vi "XML - Get relative RT Driver VI path.vi"(7 "Target Type (Windows)":T1, 10 "CD Template":refnum<class "NIVS_CD Template.lvclass">, 11 "Project Name":string) -> (3 "Relative RT Driver VI path":path)   [LabVIEW 2020, in "NIVS_Consolidated_CDW_MetaDataObj.lvclass"]
doc: "Create the relative path for the RT Driver VI inside the Configuration LLB based on the name and execution mode of the new custom device."
uses:
  NIVS_Consolidated_CDW_MetaDataObj.lvclass
  Build Spec Engine.ctl
  CD Engine lvlib.ctl
  Template Classes/NIVS_PPLCD Template/NIVS_PPLCD Template.lvclass
  Template Classes/NIVS_CD Template/NIVS_CD Template.lvclass
  Build Spec Engine.vi
  CD Engine lvlib.vi
  Target Type.ctl
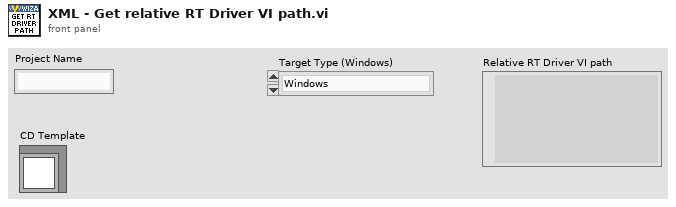
[diagram p1: front panel]
types:
  T1 = typedef "NIVS_Consolidated_CDW_MetaDataObj.lvclass/Target Type.ctl" = enum16{"Windows", "Linux x64"}
  T2 = typedef "NIVS_Consolidated_CDW_MetaDataObj.lvclass/CD Engine lvlib.ctl" = enum16{"LibraryFileName", "LibraryFolderName", "Engine.FolderName", "Engine.Init.FolderName", "Engine.Run.FolderName", "Engine.Shutdown.FolderName", "Types.FolderName", "Engine.RT Driver VI.TemplatePath", "Engine.RT Driver VI.FileName", "Engine.PPL.RT Driver VI_InlineAsync.FileName", "Engine.RTStateVariables.Name", "Engine.PPL.RTStateVariables.Name", "Engine.RTStateVariables.Name.NoExtension", "Engine.Async.NameExtension", "Engine.Async.TemplateName", "Engine.PPL.Async.TemplateName", "Engine.PPL.Async.InitVSGlobals.Name", "Engine.PPL.RT Driver VI_Inline.FileName"}
  T3 = typedef "NIVS_Consolidated_CDW_MetaDataObj.lvclass/Build Spec Engine.ctl" = enum16{"Destinations.LLBWindowsFileName", "Destinations.LLBLinux64FileName", "Destinations.PPLWindowsFileName", "Destinations.PPLLinux64FileName"}
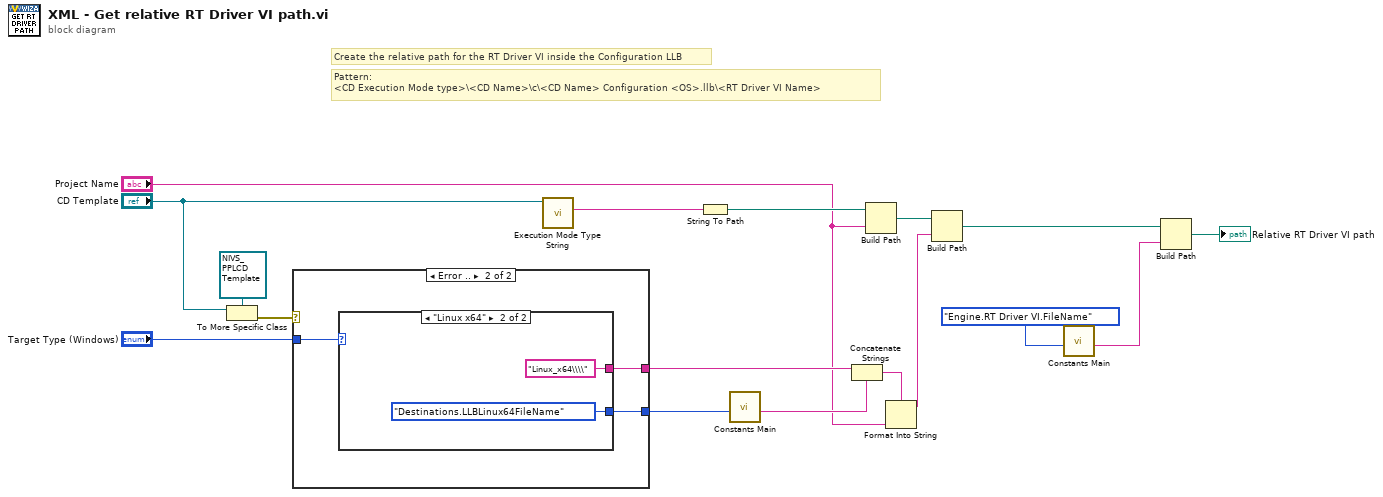
[diagram p0: block diagram]
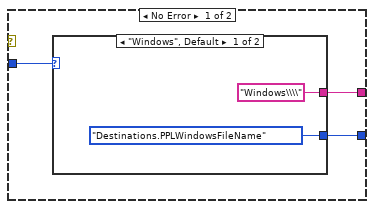
[diagram p2: hidden frame]
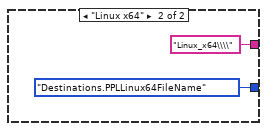
[diagram p3: hidden frame]
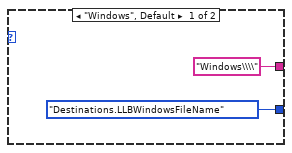
[diagram p4: hidden frame]
diagram:
  # "Create the relative path for the RT Driver VI inside the Configuration LLB"
  # "Pattern:\n<CD Execution Mode type>\\<CD Name>\\c\\<CD Name> Configuration <OS>.llb\\<RT Driver VI Name>"
  n1 = To More Specific Class(target class=refnum<class "NIVS_PPLCD Template.lvclass"> refnum ("NIVS_PPLCD Template.lvclass"), reference="CD Template") -> (error out=w1:errorcluster)  [unwired: 1 in, 1 out]
  n2 = case shown="Error .." w1 {
    tunnel: "Target Type (Windows)" -> [w18 w27]
    tunnel: [w19 w26] -> w9
    tunnel: [w20 w25] -> w6
    frame No Error {
      n3 = case shown="\"Windows\", Default" w18 {
        tunnel: [Build_Spec_Engine."Destinations.PPLWindowsFileName" ("Action") Build_Spec_Engine."Destinations.PPLLinux64FileName" ("Action")] -> w19
        tunnel: ["Windows\\\\" ("format string") "Linux_x64\\\\" ("format string")] -> w20
        frame "Windows", Default {
        }
        frame "Linux x64" {
        }
      }
    }
    frame Error {
      n4 = case shown="\"Linux x64\"" w27 {
        tunnel: [Build_Spec_Engine."Destinations.LLBWindowsFileName" ("Action") Build_Spec_Engine."Destinations.LLBLinux64FileName" ("Action")] -> w26
        tunnel: ["Windows\\\\" ("format string") "Linux_x64\\\\" ("format string")] -> w25
        frame "Windows", Default {
        }
        frame "Linux x64" {
        }
      }
    }
  }
  n5 = call-dynamic "Execution Mode Type String.vi"("CD Template"="CD Template") -> ("Execution Mode Type String"=w4:string)  [unwired: 10 in]
  n6 = String To Path(string=w4) -> (path=w14:path)
  n7 = call-poly "Constants Main.vi"("Action"=w9) -> ("Output"=w8:string)  [unwired: 10 in]
  n8 = Concatenate Strings(w6, w8) -> (w7:string)
  n9 = Build Path(base path=w14, name or relative path="Project Name") -> (appended path=w13:path)
  n10 = Format Into String(format string=w7, "Project Name") -> (resulting string=w15:string)  [unwired: 2 in, 1 out]
  n11 = Build Path(base path=w13, name or relative path=w15) -> (appended path=w11:path)
  n12 = call-poly "Constants Main.vi"("Action"=CD_Engine_lvlib."Engine.RT Driver VI.FileName") -> ("Output"=w10:string)  [unwired: 10 in]
  n13 = Build Path(base path=w11, name or relative path=w10) -> (appended path=→"Relative RT Driver VI path":path)
